vi "ArrayRemove.vi"   [LabVIEW 2009]
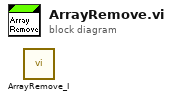
[diagram p0: block diagram]
diagram:
  n1 = call "ArrayRemove_I.vi"() -> ()  [unwired: 10 in, 2 out]
